vi "Set Output Line.vi"(8 "Error In":errorcluster, 9 "Line":i32, 10 "Value":bool, 11 "BNT_DAQmx-MCSV in":refnum<class "BNT_DAQmx-MCSV.lvclass">) -> (0 "Error Out":errorcluster, 3 "BNT_DAQmx-MCSV out":refnum<class "BNT_DAQmx-MCSV.lvclass">)   [LabVIEW 2020, in "BNT_DAQmx.lvlib" / "BNT_DAQmx-MCSV.lvclass"]
doc: "Write line value to DAQmx device and publish.\n\nTimeout is set to constant 1s."
uses:
  BNT_DAQmx-MCSV.lvclass
  BNT_DAQmx-MCSV.lvclass/BNT_DAQmx-MCSV.ctl
  <vilib>/DAQmx/write.llb/DAQmx Write (Digital 1D Bool 1Chan 1Samp).vi
  <vilib>/DAQmx/miscellaneous.llb/DAQmx Fill In Error Info.vi
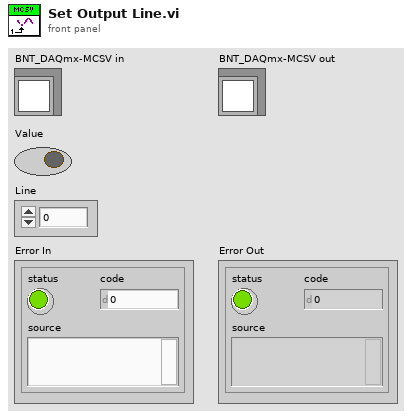
[diagram p1: front panel]
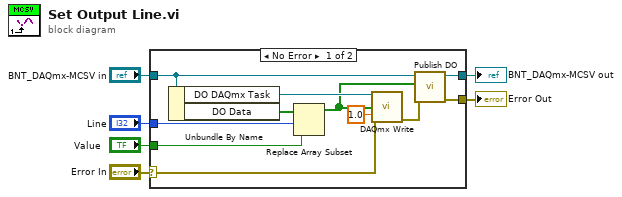
[diagram p0: block diagram]
diagram:
  n1 = case shown="No Error" "Error In" {
    selector: "Error In" -> [w15 w19]
    tunnel: [w8 w19] -> w5
    tunnel: [w7 w18] -> w3
    tunnel: "BNT_DAQmx-MCSV in" -> [w11 w18]
    tunnel: "Value" -> [w12 _]
    tunnel: "Line" -> [w13 _]
    frame No Error {
      n2 = Unbundle By Name(w11) -> ("DO DAQmx Task"=w17:refnum<k21>, "DO Data"=w14:bool[])
      n3 = Replace Array Subset(array=w14, new element=w12, index=w13) -> (w10:bool[])
      n4 = call-poly <vilib>:"DAQmx Write.vi"("task/channels in"=w17, "data"=w10, "timeout"=1.0, "error in"=w15) -> ("error out"=w9:errorcluster)  [unwired: 9 in, 2 out]
      n5 = call "Publish DO.vi"("error in"=w9, "DO Data"=w10, "BNT_DAQmx-MCSV in"=w11) -> ("error out"=w8:errorcluster, "BNT_DAQmx-MCSV out"=w7:refnum<class "BNT_DAQmx-MCSV.lvclass">)  [unwired: 7 in]
    }
    frame Error {
    }
  }
  "Error Out" <- w5
  "BNT_DAQmx-MCSV out" <- w3
